vi "__uintPow.vi"(8 "Base (decimal)":T1=10 items=["Binary"=2, "Octal"=8, "Decimal"=10, "Hexadecimal"=16, "Hexatrigesimal"=36, "ASCII"=64], 10 "Exponent (2)":u32=2, 11 "UInt in":u8[](array[numeric])=[0]) -> (0 "Timing multiplication":u32, 3 "UInt^Exponent":u8[](array[numeric]))   [LabVIEW 2011, in "UintClass.lvclass"]
uses:
  UintClass.lvclass
  enumBase.ctl
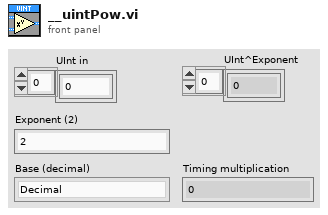
[diagram p1: front panel]
types:
  T1 = typedef "UintClass.lvclass/enumBase.ctl" = u16
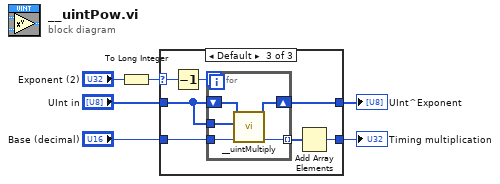
[diagram p0: block diagram]
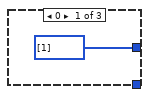
[diagram p2: hidden frame]
diagram:
  n1 = To Long Integer(number="Exponent (2)") -> (32bit integer=w1:i32)
  n2 = case shown="Default" w1 {
    selector: w1 -> [_ _ w10]
    tunnel: [u8[] [1] ("UInt in") w8 w15] -> w6
    tunnel: "Base (decimal)" -> [_ _ w14]
    tunnel: "UInt in" -> [_ w8 w13]
    tunnel: [_ _ w11] -> w3
    frame 0 {
    }
    frame 1 {
    }
    frame Default {
      n3 = Decrement(x=w10) -> (x-1=w9:i32)
      n4 = for {
        N: w9 -> [_]
        tunnel: w14 -> [w18]
        tunnel: w13 -> [w19]
        shift-right: [w16] -> w15
        shift-left: w13 -> [w20]
        tunnel: [w17] -> w12 mode=indexing
        n5 = call "__uintMultiply.vi"("Base (decimal)"=w18, "UInt2 in"=w19, "UInt1 in"=w20) -> ("Timing multiplication"=w17:u32, "UInt1 * Uint2"=w16:u8[])  [unwired: 7 in]
      }
      n6 = Add Array Elements(numeric array=w12) -> (sum=w11:u32)
    }
  }
  "Timing multiplication" <- w3
  "UInt^Exponent" <- w6
